vi "working_interface.vi"() -> ()   [LabVIEW 2011]
panel:
  out "Digital Waveform Graph":digitalwaveform(graph)
  in  "read delay data":bool
  in  "write command?":bool
  in  "command":string="*TRG"
  in  "VISA resource name":refnum<visa-resource-name>
  out "error out":errorcluster
  in  "stop":bool
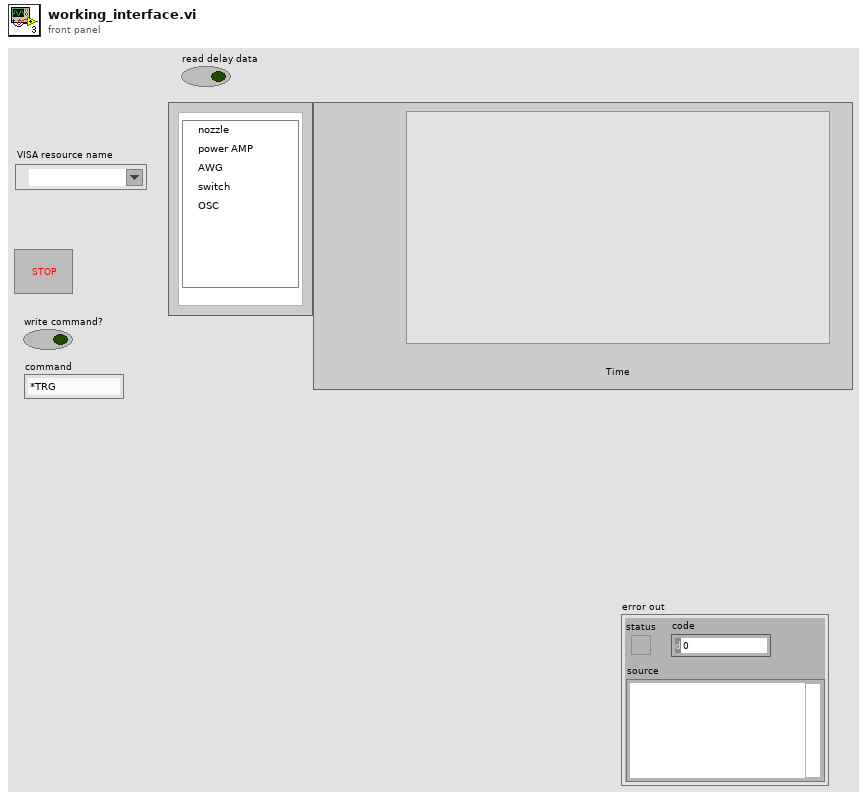
[diagram p1: front panel]
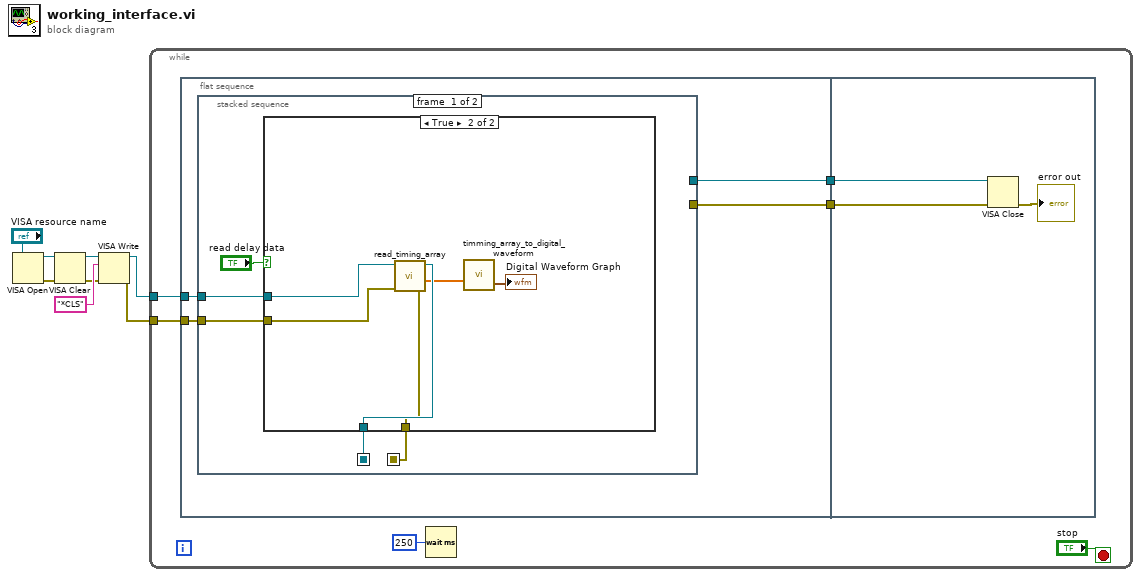
[diagram p0: block diagram]
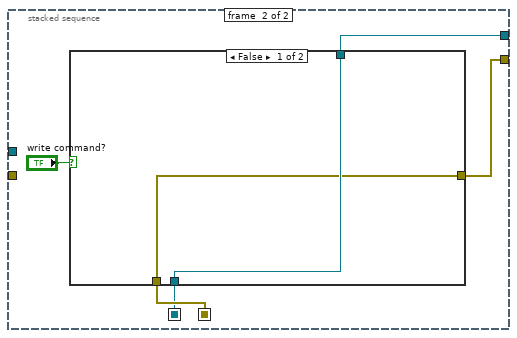
[diagram p3: hidden frame]
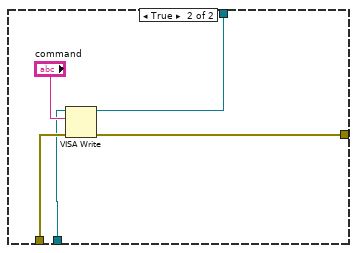
[diagram p4: hidden frame]
diagram:
  n1 = VISA Open(VISA resource name="VISA resource name") -> (VISA resource name=w5:refnum<visa-resource-name>, error out=w6:errorcluster)  [unwired: 4 in]
  n2 = VISA Clear(VISA resource name=w5, error in (no error)=w6) -> (VISA resource name out=w2:refnum<visa-resource-name>, error out=w1:errorcluster)
  n3 = VISA Write(VISA resource name=w2, write buffer="*CLS" ("Query 2"), error in (no error)=w1) -> (VISA resource name out=w4:refnum<visa-resource-name>, error out=w3:errorcluster)  [unwired: 1 out]
  n4 = while {
    tunnel: w4 -> [w10]
    tunnel: w3 -> [w9]
    stop <- "stop" stop-if-true
    n5 = flat-sequence {
      tunnel: [w16] -> w12
      tunnel: [w15] -> w11
      tunnel: w9 -> [w17]
      tunnel: w10 -> [w18]
      tunnel: w12 -> [w45]
      tunnel: w11 -> [w44]
      frame #0 {
        n6 = stacked-sequence {
          seq-local: [w21 _] -> [_ w35]
          seq-local: [w20 _] -> [_ w36]
          tunnel: w18 -> [w23 _]
          tunnel: w17 -> [w22 _]
          tunnel: [_ w33] -> w16
          tunnel: [_ w34] -> w15
          frame #0 {
            n7 = case shown="True" "read delay data" {
              tunnel: w23 -> [w24 w31]
              tunnel: w22 -> [w25 w30]
              tunnel: [w24 w29] -> w21
              tunnel: [w25 w28] -> w20
              frame False {
              }
              frame True {
                n8 = call "read_timing_array.vi"("error in"=w30, "VISA resource in"=w31) -> ("error out 2"=w28:errorcluster, "delay array"=w27:dbl[], "VISA resource out"=w29:refnum<visa-resource-name>)  [unwired: 3 in]
                n9 = call "timming_array_to_digital_waveform.vi"("timing array"=w27) -> ("digital waveform"=→"Digital Waveform Graph":digitalwaveform)  [unwired: 3 in]
              }
            }
          }
          frame #1 {
            n10 = case shown="False" "write command?" {
              tunnel: w36 -> [w37 w42]
              tunnel: w35 -> [w38 w41]
              tunnel: [w38 w40] -> w34
              tunnel: [w37 w39] -> w33
              frame False {
              }
              frame True {
                n11 = VISA Write(VISA resource name=w41, write buffer="command", error in (no error)=w42) -> (VISA resource name out=w40:refnum<visa-resource-name>, error out=w39:errorcluster)  [unwired: 1 out]
              }
            }
          }
        }
      }
      frame #1 {
        n12 = VISA Close(VISA resource name=w44, error in (no error)=w45) -> (error out=→"error out":errorcluster)
      }
    }
    n13 = Wait (ms)(milliseconds to wait=u32 250) -> ()  [unwired: 1 out]
  }
